vi "AO Array Add or Remove.vi"(8 "error in (no error)":errorcluster, 10 "Size":i32, 11 "AO Channels in":T1 {"Phase" format="%.3g"; "Frequency" min=0.0001 max=10000.0 format="%.3g"; "Offset" format="%.3p"; "Amplitude" min=0.0 max=10.0 format="%.3p"}) -> (0 "error out":errorcluster, 3 "AO Channels out":T1 {"Phase" format="%.3g"; "Frequency" min=0.0001 max=10000.0 format="%.3g"; "Offset" format="%.3p"; "Amplitude" min=0.0 max=10.0 format="%.3p"})   [LabVIEW 2019, in "Instrument.DAQ.lvclass"]
uses:
  Instrument.DAQ.lvclass
  Typedefs/AO.Channel--Cluster--Array.ctl
  Typedefs/AO.Channel--Cluster.ctl
  Typedefs/AO.Channel.Function--Enum.ctl
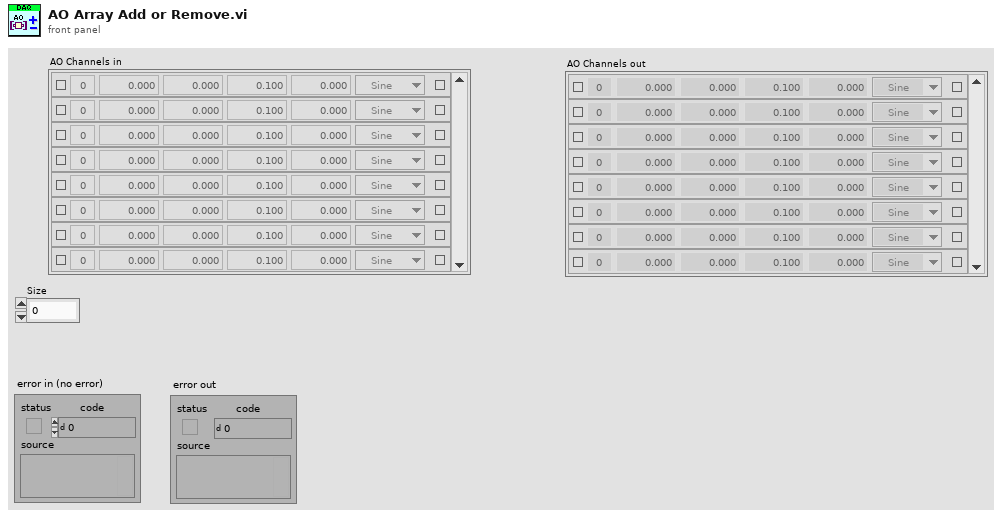
[diagram p1: front panel]
types:
  T1 = typedef "Instrument.DAQ.lvclass/AO.Channel--Cluster--Array.ctl" = T2[]
  T2 = typedef "Instrument.DAQ.lvclass/AO.Channel--Cluster.ctl" = cluster{"Enable?":bool, "Channel":i32, "Amplitude":dbl, "Offset":dbl, "Frequency":dbl, "Phase":dbl, "Function":T3, "Sweeping?":bool}
  T3 = typedef "Instrument.DAQ.lvclass/AO.Channel.Function--Enum.ctl" = enum16{"Sine", "Triangle", "Square"}
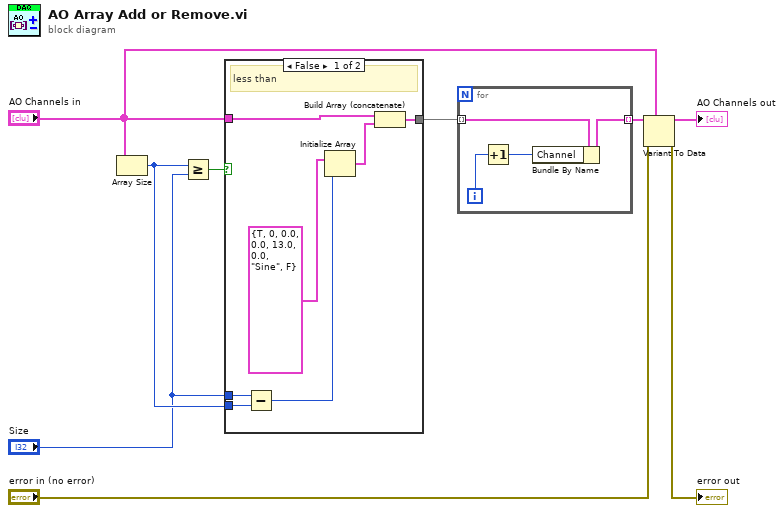
[diagram p0: block diagram]
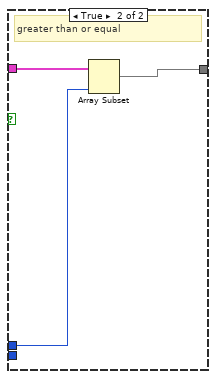
[diagram p2: hidden frame]
diagram:
  n1 = Array Size(array="AO Channels in") -> (size(s)=w9:i32)
  n2 = Greater Or Equal?(x=w9, y="Size") -> (x >= y?=w8:bool)
  n3 = case shown="False" w8 {
    tunnel: "AO Channels in" -> [w11 w19]
    tunnel: "Size" -> [w14 w18]
    tunnel: [w15 w17] -> w7
    tunnel: w9 -> [w13 _]
    frame False {
      # "less than"
      n4 = Subtract(x=w14, y=w13) -> (x-y=w12:i32)
      n5 = Initialize Array(T2 {"Enable?"=TRUE, "Channel"=0, "Amplitude"=0.0, "Offset"=0.0, "Frequency"=13.0, "Phase"=0.0, "Function"=enum."Sine", "Sweeping?"=FALSE} ("AO"), w12) -> (w16:T2[])
      n6 = Build Array (concatenate)(w11, w16) -> (w15:T1)
    }
    frame True {
      # "greater than or equal"
      n7 = Array Subset(array=w19, length=w18) -> (w17:T1)  [unwired: 1 in]
    }
  }
  n8 = for {
    tunnel: w7 -> [w23] mode=indexing
    tunnel: [w22] -> w5 mode=indexing
    i -> [w20]
    n9 = Increment(x=w20) -> (x+1=w21:i32)
    n10 = Bundle By Name(cluster=w23, "Channel"=w21) -> (w22:T2)
  }
  n11 = Variant To Data(error in="error in (no error)", type="AO Channels in", Variant=w5) -> (data=→"AO Channels out":T1, error out=→"error out":errorcluster)
